vi "Build Array.vi"(8 "error in (no error)":errorcluster, 10 "1D array":dbl[](array[numeric]), 11 "initialized 2D in":dbl[][](array[numeric])) -> (0 "error out":errorcluster, 3 "initialized 2D out":dbl[][](array[numeric]))   [LabVIEW 2015, in "Zen Analytics.lvlib" / "Zen Analytics.lvclass"]
uses:
  Zen Analytics.lvclass
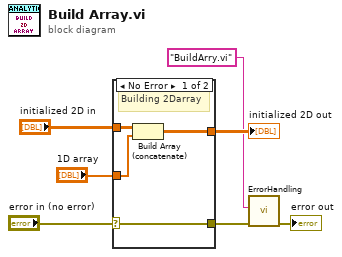
[diagram p0: block diagram]
diagram:
  n1 = case shown="No Error" "error in (no error)" {
    selector: "error in (no error)" -> [w11 w13]
    tunnel: [w11 w13] -> w2
    tunnel: "initialized 2D in" -> [w10 w12]
    tunnel: "1D array" -> [w9 _]
    tunnel: [w8 w12] -> w4
    frame No Error {
      # "Building 2Darray"
      n2 = Build Array (concatenate)(w10, w9) -> (w8:dbl[][])
    }
    frame Error {
    }
  }
  "initialized 2D out" <- w4
  n3 = call "ErrorHandling.vi"("error in (no error)"=w2, "Vi-name"="BuildArry.vi") -> ("error out"=→"error out":errorcluster)  [unwired: 9 in]
